vi "MovimientoMonocromador.vi"(8 "comenzar":bool, 10 "destino":dbl, 11 "actual":dbl) -> (2 "longitud actual":dbl)   [LabVIEW 2016]
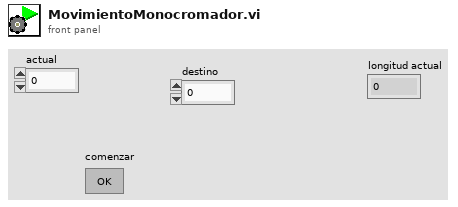
[diagram p1: front panel]
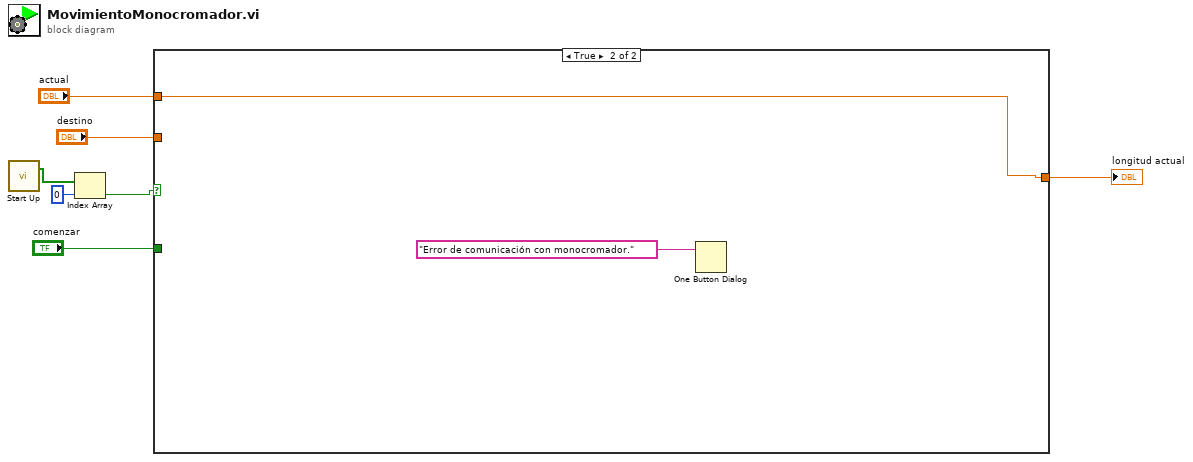
[diagram p0: block diagram]
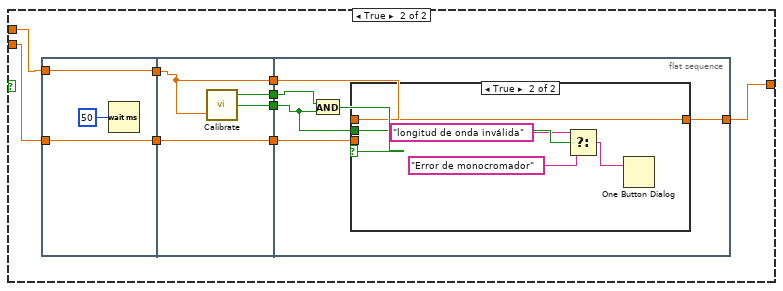
[diagram p3: hidden frame]
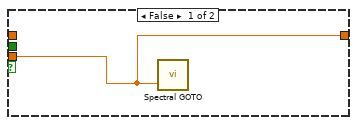
[diagram p4: hidden frame]
diagram:
  n1 = call "Start Up.VI"() -> ("Error List"=w7:bool[])  [unwired: 1 in, 1 out]
  n2 = Index Array(array=w7, index=0) -> (element=w5:bool)
  n3 = case shown="True" w5 {
    tunnel: "destino" -> [w9 _]
    tunnel: "actual" -> [w10 w41]
    tunnel: "comenzar" -> [w11 _]
    tunnel: [w8 w41] -> w1
    frame False {
      n4 = case shown="False" w11 {
        tunnel: w10 -> [w12 w21]
        tunnel: w9 -> [_ w15]
        tunnel: [w12 w14] -> w8
        frame False {
        }
        frame True {
          n5 = flat-sequence {
            tunnel: w21 -> [w23]
            tunnel: [w23] -> w20
            tunnel: w15 -> [w22]
            tunnel: [w22] -> w17
            tunnel: w20 -> [w25]
            tunnel: [w28] -> w19
            tunnel: [w27] -> w18
            tunnel: w17 -> [w26]
            tunnel: [w26] -> w16
            tunnel: [w25] -> w13
            tunnel: w19 -> [w34]
            tunnel: w18 -> [w29]
            tunnel: w16 -> [w32]
            tunnel: [w31] -> w14
            tunnel: w13 -> [w30]
            frame #0 {
              n6 = Wait (ms)(milliseconds to wait=u32 50) -> ()  [unwired: 1 out]
            }
            frame #1 {
              n7 = call "Calibrate.VI"("Counter Position"=w25) -> ("Error"=w28:bool, "Invalid Wavelength"=w27:bool)  [unwired: 1 in, 1 out]
            }
            frame #2 {
              n8 = And(x=w34, y=w29) -> (x .and. y?=w33:bool)
              n9 = case shown="True" w33 {
                tunnel: w32 -> [w35 _]
                tunnel: [w35 w40] -> w31
                tunnel: w30 -> [_ w40]
                tunnel: w29 -> [_ w38]
                frame False {
                  n10 = call "Spectral GOTO.VI"("Target Position"=w35) -> ()  [unwired: 1 in, 3 out]
                }
                frame True {
                  n11 = Select(t="longitud de onda inválida", s=w38, f="Error de monocromador" ("message")) -> (s? t:f=w37:string)
                  n12 = One Button Dialog(message=w37) -> ()  [unwired: 1 in, 1 out]
                }
              }
            }
          }
        }
      }
    }
    frame True {
      n13 = One Button Dialog(message="Error de comunicación con monocromador.") -> ()  [unwired: 1 in, 1 out]
    }
  }
  "longitud actual" <- w1
